vi "wpisz_plik.vi"(8 "error in":errorcluster, 11 "HR Data Structure":T1={"Runer's Data"={"Name"="", "Age"=0}, "HR Max"=0, "Raw Data"={"Time"=[], "Bpm"=[]}, "% HR MAX "=[], "HR Zones "=[], "no of points"=[], "Heart Rate Zone No 2"=[1, 2, 3, 4, 5], "History"=[["training number", "HR Max value", "HR Mean value"], ["", "", ""]], "number history"=0}) -> (0 "error out":errorcluster, 2 "text":string, 3 "HR Data Structure 2":T1={"Runer's Data"={"Name"="", "Age"=0}, "HR Max"=0, "Raw Data"={"Time"=[], "Bpm"=[]}, "% HR MAX "=[], "HR Zones "=[], "no of points"=[], "Heart Rate Zone No 2"=[1, 2, 3, 4, 5], "History"=[["training number", "HR Max value", "HR Mean value"], ["", "", ""]], "number history"=0})   [LabVIEW 2024]
uses:
  zad_3-labview/klaster 4.ctl
  zad_3-labview/klaster.ctl
  zad_3-labview/klaster 2.ctl
panel:
  out "String":string
  in  "Button":bool
  in  "?":path
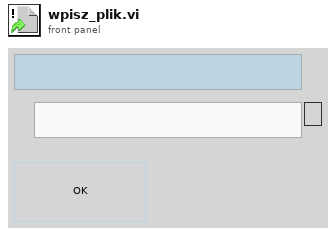
[diagram p1: front panel]
types:
  T1 = typedef "klaster 4.ctl" = cluster{"Runer's Data":T2, "HR Max":i32, "Raw Data":T3, "% HR MAX ":dbl[], "HR Zones ":string[][], "no of points":dbl[], "Heart Rate Zone No 2":i32[], "History":string[][], "number history":i32}
  T2 = typedef "klaster.ctl" = cluster{"Name":string, "Age":i32}
  T3 = typedef "klaster 2.ctl" = cluster{"Time":timestamp[], "Bpm":i32[]}
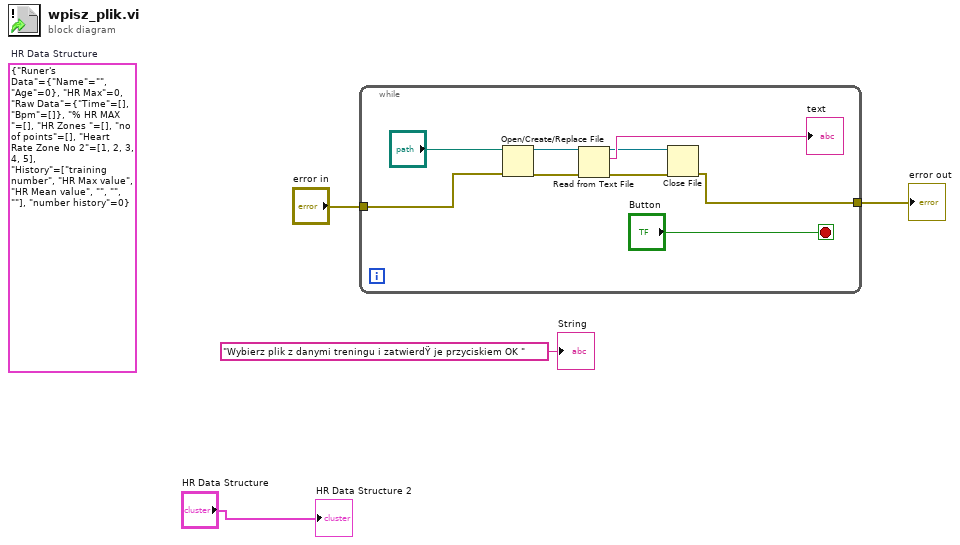
[diagram p0: block diagram]
diagram:
  (unwired) T1 {"Runer's Data"={"Name"="", "Age"=0}, "HR Max"=0, "Raw Data"={"Time"=[], "Bpm"=[]}, "% HR MAX "=[], "HR Zones "=[], "no of points"=[], "Heart Rate Zone No 2"=[1, 2, 3, 4, 5], "History"=[["training number", "HR Max value", "HR Mean value"], ["", "", ""]], "number history"=0}  # HR Data Structure
  n1 = while {
    tunnel: "error in" -> [w6]
    tunnel: [w5] -> w2
    stop <- "Button" stop-if-true
    n2 = Open/Create/Replace File(file path (use dialog)="?", error in=w6) -> (refnum out=w12:refnum<file>, error out=w11:errorcluster)  [unwired: 4 in, 1 out]
    n3 = Read from Text File(file (use dialog)=w12, error in=w11) -> (refnum out=w9:refnum<file>, text=→"text":string, error out=w10:errorcluster)  [unwired: 2 in, 1 out]
    n4 = Close File(refnum=w9, error in=w10) -> (error out=w5:errorcluster)  [unwired: 1 out]
  }
  "error out" <- w2
  "HR Data Structure 2" <- "HR Data Structure"
  "String" <- "Wybierz plik z danymi treningu i zatwierdŸ je przyciskiem OK " ("String")
